vi "Verificacion_calibracion.vi"() -> ()   [LabVIEW 2015]
uses:
  <vilib>/LabVIEW Targets/FPGA/cRIO/shared/nicrio_ModuleControls/nicrio_cRIO-9234_DataRatesRing2.ctl
  <vilib>/userdefined/High Color/nirio_resource_hc.ctl
  <vilib>/Analysis/5stat.llb/RMS (DBL).vi
  <vilib>/Analysis/baseanly.llb/Mean (DBL).vi
  <vilib>/FPGAPlugInAG/cRIO-9031/niLvFpga_Open_cRIO-9031.vi
  <vilib>/FPGAPlugInAG/cRIO-9031/niLvFpga_Run_cRIO-9031.vi
  <vilib>/Utility/error.llb/Error Cluster From Error Code.vi
  <vilib>/rvi/errors/niLvFpgaAdjustHostInterfaceError.vi
  <vilib>/rvi/interface/common/niFpgaWaitOnOcc.vi
  <vilib>/FPGAPlugInAG/cRIO-9031/niLvFpga_Reset_cRIO-9031.vi
  <vilib>/measure/madcrms.llb/Basic Averaged DC-RMS for 1 Chan.vi
  <vilib>/measure/maspectr.llb/FFT Spectrum (Mag-Phase) for 1 Chan.vi
  <vilib>/FPGAPlugInAG/cRIO-9031/niLvFpga_Close_cRIO-9031.vi
  <vilib>/rvi/interface/nirviOpenFPGA/nirviOpenFPGA.xnode
  FPGA Bitfiles/WRDArabia_FPGATarget_FPGA8a2wsBIdirec_rZEOcJD8nrk.lvbitx
  <vilib>/rvi/interface/nirviMethod/nirviMethod.xnode
  <vilib>/rvi/interface/nirviReadWriteControl/nirviReadWriteControl.xnode
  <vilib>/rvi/interface/nirviCloseFPGA/nirviCloseFPGA.xnode
  <vilib>/measure/NI_MAPro.lvlib
  <vilib>/Analysis/NI_AALPro.lvlib
  <vilib>/Analysis/NI_AALBase.lvlib
  <vilib>/rvi/errors/niLvFpgaMergeErrorWithErrorCode.vi
  NiFpgaLv.dll
  <vilib>/FPGAPlugInAG/cRIO-9031/niLvFpga_ConfigureFifo_cRIO-9031.vi
  <vilib>/FPGAPlugInAG/cRIO-9031/niLvFpga_StartFifo_cRIO-9031.vi
  <vilib>/FPGAPlugInAG/cRIO-9031/niLvFpga_ReadFifo_cRIO-9031.vi
  <vilib>/FPGAPlugInAG/cRIO-9031/niLvFpga_StopFifo_cRIO-9031.vi
panel:
  out "size(s)":i32
  out "Numeric":i32
  in  "Pattern acceleration (g RMS)":dbl=1.0
  in  "Pattern frequency (Hz)":dbl=159.2
  out "RMS":dbl format="%0.2f"
  in  "Data Rate":T1=2 items=["51.200 kS/s (NI 9234)"=1, "25.600 kS/s (NI 9234)"=2, "17.067 kS/s (NI 9234)"=3, "12.800 kS/s (NI 9234)"=4, "10.240 kS/s (NI 9234)"=5, "8.533 kS/s (NI 9234)"=6, "7.314 kS/s (NI 9234)"=7, "6.400 kS/s (NI 9234)"=8, "5.689 kS/s (NI 9234)"=9, "5.120 kS/s (NI 9234)"=10, "4.654 kS/s (NI 9234)"=11, "4.267 kS/s (NI 9234)"=12, "3.938 kS/s (NI 9234)"=13, "3.657 kS/s (NI 9234)"=14, "3.413 kS/s (NI 9234)"=15, "3.200 kS/s (NI 9234)"=16, "3.012 kS/s (NI 9234)"=17, "2.845 kS/s (NI 9234)"=18, "2.695 kS/s (NI 9234)"=19, "2.560 kS/s (NI 9234)"=20, "2.438 kS/s (NI 9234)"=21, "2.328 kS/s (NI 9234)"=22, "2.226 kS/s (NI 9234)"=23, "2.133 kS/s (NI 9234)"=24, "2.048 kS/s (NI 9234)"=25, "1.969 kS/s (NI 9234)"=26, "1.896 kS/s (NI 9234)"=27, "1.829 kS/s (NI 9234)"=28, "1.765 kS/s (NI 9234)"=29, "1.707 kS/s (NI 9234)"=30, "1.652 kS/s (NI 9234)"=31]
  in  "Channel Nº":i32
  out "FREQUENCY SIGNAL":cluster{"f0":dbl, "df":dbl, "magnitude":dbl[]}(graph)
  out "error out":errorcluster
  out "Chassis \nTemperature":i16
  in  "Adquirir":bool
  out "Waveform Graph":waveform(dbl)[](graph)
  out "Frequency measured (Hz)":dbl
  in  "Sensivity Parameter\n           (mV/g)":sgl=10.0
  in  "Rate frequency (Hz)":dbl=25600.0
  in  "Calibration channels (4 o 8)":u32=8
  out "Nombre de archivo":path
  out "Tiempo de paso (s)":dbl
  in  "Acquisition time":dbl=1.0
  out "Buffer Overflow":bool
  out "Buffer Underflow":bool
  in  "stop":bool
  out "Inicio pasada":timestamp
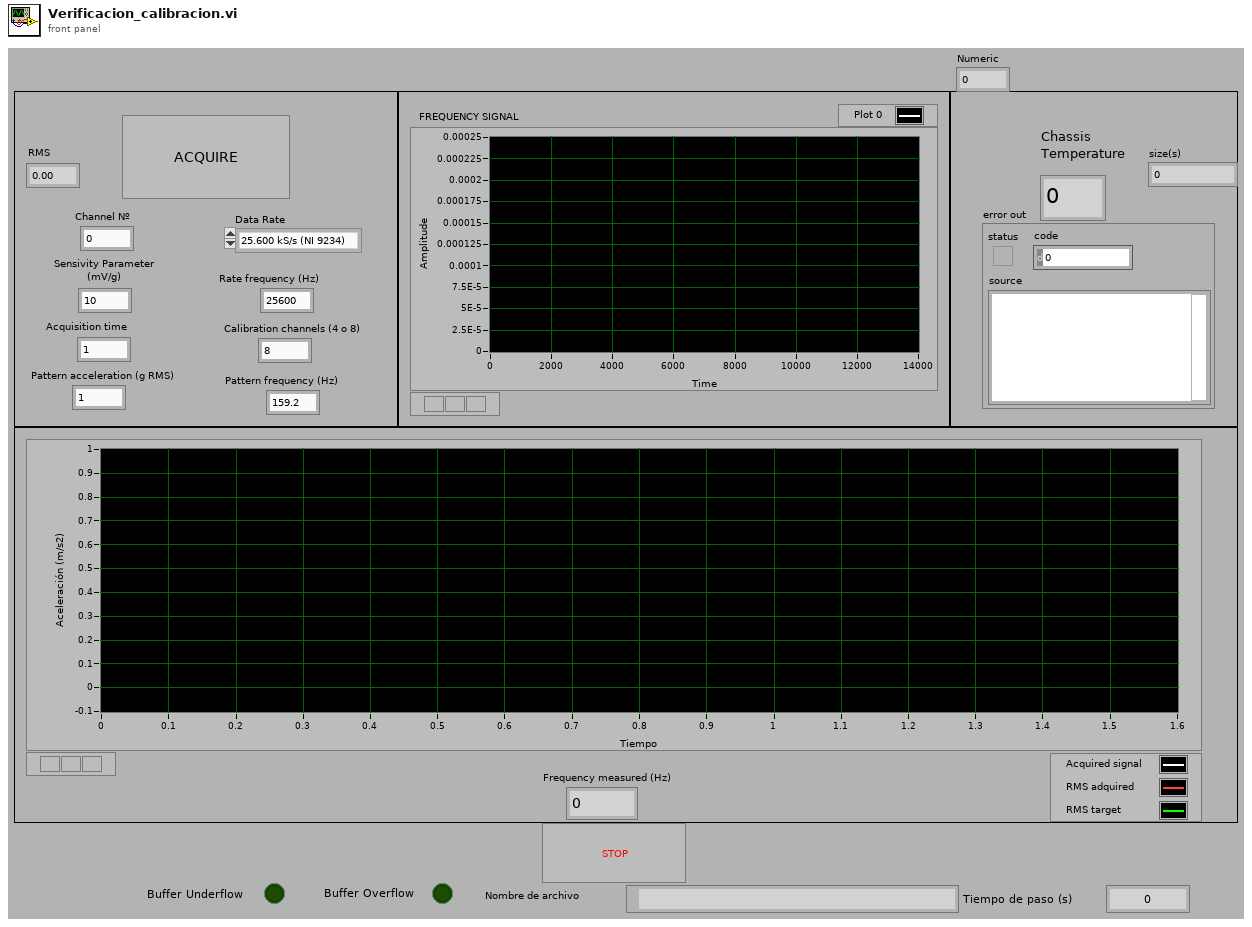
[diagram p1: front panel]
types:
  T1 = typedef "nicrio_cRIO-9234_DataRatesRing2.ctl" = u8
  T2 = typedef "nirio_resource_hc.ctl" = tag
  T3 = enum16{"open", "replace", "create", "open or create", "replace or create", "replace or create with confirmation"}
  T4 = enum16{"big-endian, network order", "native, host order", "little-endian"}
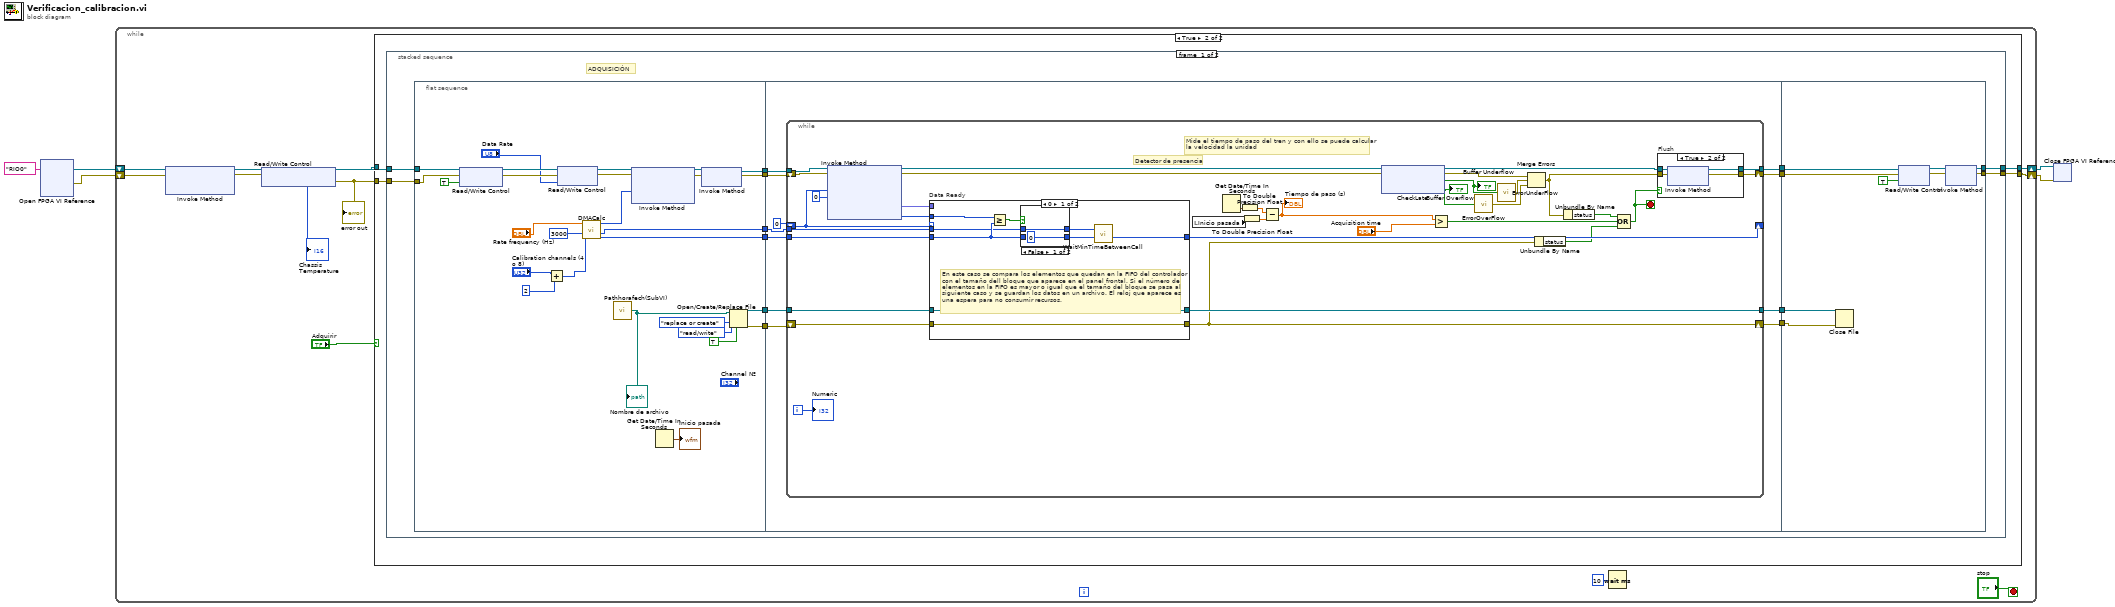
[diagram p0: block diagram]
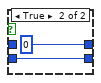
[diagram p3: hidden frame]
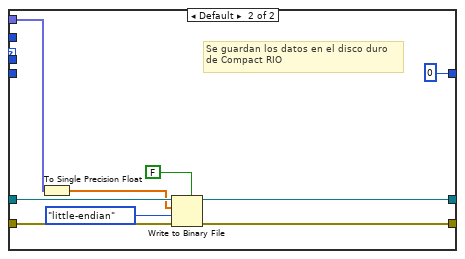
[diagram p4: hidden frame]
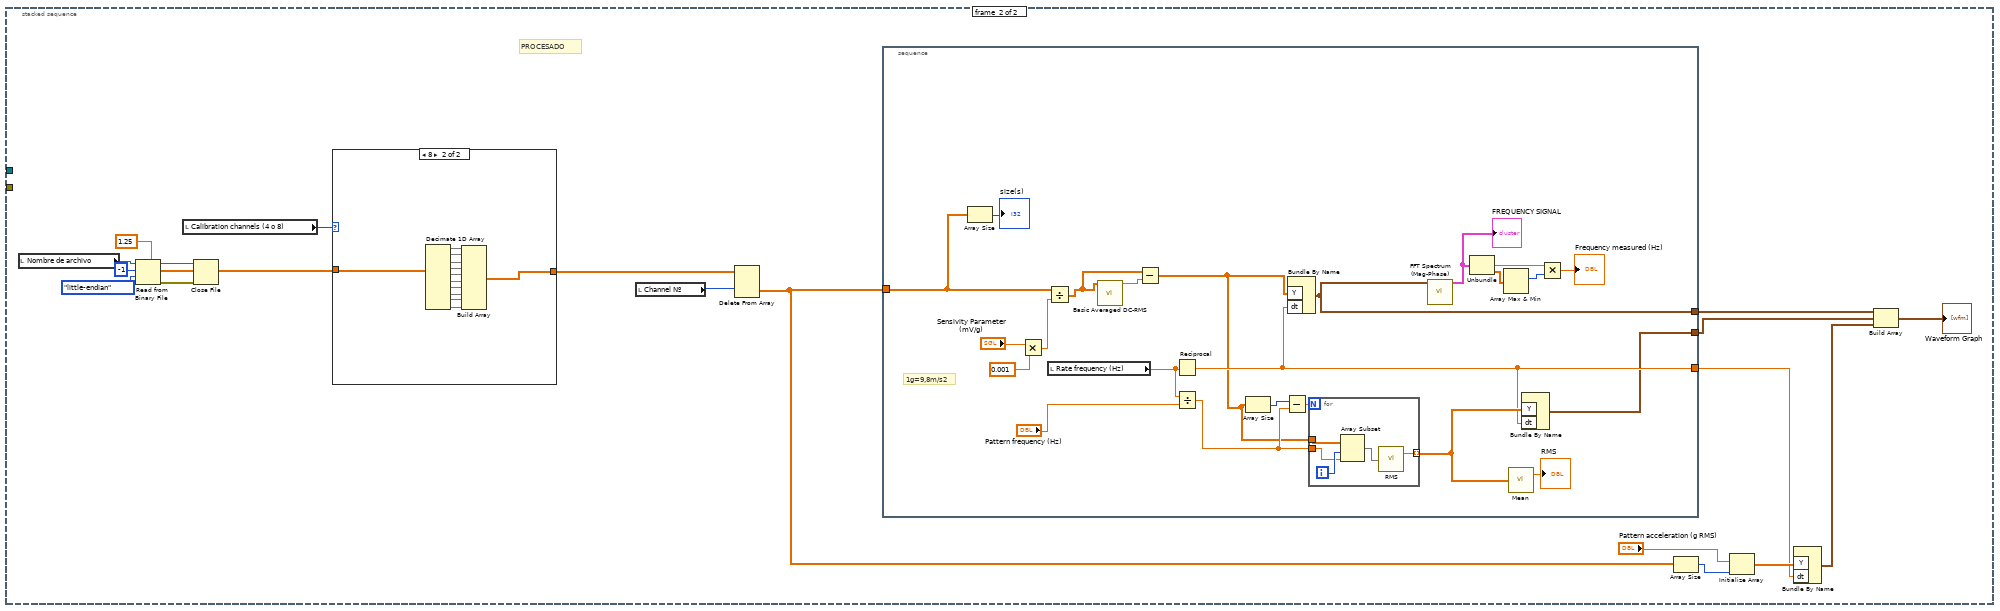
[diagram p6: hidden frame]
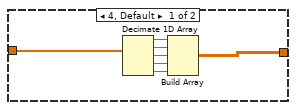
[diagram p7: hidden frame]
diagram:
  n1 = xnode "Open FPGA VI Reference"("resource name"=T2 "RIO0") -> ("FPGA VI Reference Out"=w5:refnum<k20>, "error out"=w2:errorcluster)  [unwired: 1 in]
  n2 = while {
    shift-right: [w10] -> w3
    shift-left: w5 -> [w8]
    shift-right: [w15] -> w4
    shift-left: w2 -> [w7]
    stop <- "stop" stop-if-true
    n3 = xnode "Invoke Method"("FPGA VI Reference In"=w8, "error in"=w7) -> ("FPGA VI Reference Out"=w9:refnum<k20>, "error out"=w6:errorcluster)  [unwired: 1 in]
    n4 = xnode "Read/Write Control"("FPGA VI Reference In"=w9, "error in"=w6) -> ("FPGA VI Reference Out"=w13:refnum<k20>, "error out"=w12:errorcluster, "Chassis Temperature"=→"Chassis \nTemperature":i16)
    "error out" <- w12
    n5 = case shown="True" "Adquirir" {
      tunnel: w13 -> [w19 w23]
      tunnel: w12 -> [w18 w22]
      tunnel: [w19 w21] -> w10
      tunnel: [w18 w20] -> w15
      frame False {
      }
      frame True {
        n6 = stacked-sequence {
          tunnel: w23 -> [w27 _]
          tunnel: w22 -> [w26 _]
          tunnel: [w25 _] -> w21
          tunnel: [w24 _] -> w20
          frame #0 {
            # "ADQUISICIÓN"
            n7 = flat-sequence {
              tunnel: w26 -> [w45]
              tunnel: w27 -> [w46]
              tunnel: [w57] -> w37
              tunnel: [w56] -> w36
              tunnel: [w55] -> w35
              tunnel: [w54] -> w34
              tunnel: [w53] -> w33
              tunnel: [w52] -> w32
              tunnel: [w74] -> w31
              tunnel: [w73] -> w30
              tunnel: [w72] -> w29
              tunnel: [w65] -> w28
              tunnel: w37 -> [w71]
              tunnel: w36 -> [w70]
              tunnel: w35 -> [w69]
              tunnel: w34 -> [w68]
              tunnel: w33 -> [w67]
              tunnel: w32 -> [w66]
              tunnel: w31 -> [w139]
              tunnel: w30 -> [w138]
              tunnel: w29 -> [w144]
              tunnel: w28 -> [w143]
              tunnel: [w145] -> w24
              tunnel: [w146] -> w25
              frame #0 {
                n8 = xnode "Read/Write Control"("FPGA VI Reference In"=w46, "error in"=w45, "Fotocélula"=TRUE ("Adquirir")) -> ("FPGA VI Reference Out"=w44:refnum<k20>, "error out"=w43:errorcluster)
                n9 = Add(x="Calibration channels (4 o 8)", y=u32 2) -> (x+y=w39:u32)
                n10 = xnode "Read/Write Control"("FPGA VI Reference In"=w44, "error in"=w43, "Data Rate"="Data Rate") -> ("FPGA VI Reference Out"=w50:refnum<k20>, "error out"=w49:errorcluster)
                n11 = call "DMACalc.vi"("Number of Channels"=w39, "Number of Samples"=u32 3000, "Rate (Hz)"="Rate frequency (Hz)") -> ("Block Size"=w54:u32, "Time to Acquire Block (ms)"=w55:i32, "Host Buffer Size"=w59:u32)  [unwired: 6 in]
                n12 = call "Pathhorafech(SubVI).vi"() -> ("path"=w58:path)
                "Nombre de archivo" <- w58
                n13 = xnode "Invoke Method"("FPGA VI Reference In"=w50, "error in"=w49, "Requested Depth"=w59) -> ("FPGA VI Reference Out"=w61:refnum<k20>, "error out"=w60:errorcluster)  [unwired: 1 out]
                n14 = Get Date/Time In Seconds() -> (seconds since 1Jan1904=→"Inicio pasada":timestamp)
                n15 = xnode "Invoke Method"("FPGA VI Reference In"=w61, "error in"=w60) -> ("FPGA VI Reference Out"=w57:refnum<k20>, "error out"=w56:errorcluster)
                n16 = Open/Create/Replace File(file path (use dialog)=w58, operation (0:open)=T3."replace or create", access (0:read/write)=enum16{"read/write", "read-only", "write-only"}."read/write", disable buffering (F)=TRUE) -> (refnum out=w53:refnum<file>, error out=w52:errorcluster)  [unwired: 1 in, 2 out]
              }
              frame #1 {
                n17 = while "Data Acquisition" {
                  tunnel: w71 -> [w101]
                  shift-right: [w108] -> _
                  shift-left: u32 0 ("t") -> [w104]
                  tunnel: w69 -> [w109]
                  tunnel: w68 -> [w107]
                  shift-right: [w110] -> w73
                  shift-left: w70 -> [w100]
                  tunnel: [w105] -> w74
                  tunnel: w67 -> [w88]
                  tunnel: [w89] -> w72
                  shift-right: [w87] -> w65
                  shift-left: w66 -> [w98]
                  i -> [w76]
                  stop <- w106 stop-if-true
                  # "Detector de presencia"
                  # "Mide el tiempo de paso del tren y con ello se puede calcular\nla velocidad la unidad"
                  n18 = xnode "Invoke Method"("FPGA VI Reference In"=w101, "error in"=w100, "Number of Elements"=w104, "Timeout (ms)"=0) -> ("FPGA VI Reference Out"=w86:refnum<k20>, "error out"=w85:errorcluster, "Data"=w99:fxp<+/-,24,4>[], "Elements Remaining"=w102:u32)
                  n19 = case "Data Ready" shown="0" w104 {
                    tunnel: w109 -> [w115 _]
                    tunnel: [w114 u32 0 ("t")] -> w108
                    tunnel: w107 -> [w116 _]
                    tunnel: w102 -> [w113 _]
                    tunnel: w99 -> [_ w126]
                    tunnel: w98 -> [w112 w128]
                    tunnel: [w112 w127] -> w87
                    tunnel: w88 -> [w111 w125]
                    tunnel: [w111 w124] -> w89
                    frame 0 {
                      # "En este caso se compara los elementos que quedan en la FIFO del controlador\ncon el tamaño dell bloque que aparece en el panel frontal. Si el número de\nelementos en la FIFO es mayor o igual que el tamaño del bloque se pasa al\nsiguiente caso y se guardan los datos en un archivo. El reloj que aparece es\nuna espera para no consumir recursos."
                      n20 = Greater Or Equal?(x=w113, y=w116) -> (x >= y?=w117:bool)
                      n21 = case shown="False" w117 {
                        tunnel: [u32 0 ("Block Size") w121] -> w114
                        tunnel: [w120 0 ("t")] -> w118
                        tunnel: w115 -> [w120 _]
                        tunnel: w116 -> [_ w121]
                        frame False {
                        }
                        frame True {
                        }
                      }
                      n22 = call "WaitMinTimeBetweenCall.vi"("Minimum ms between calls"=w118) -> ()  [unwired: 2 in]
                    }
                    frame Default {
                      # "Se guardan los datos en el disco duro\nde Compact RIO"
                      n23 = To Single Precision Float(number=w126) -> (single precision float=w123:sgl[])
                      n24 = Write to Binary File(file (use dialog)=w125, data=w123, error in=w128, 5:FALSE ("prepend array or string size? (T)"), 9:T4."little-endian" ("byte order (0:big-endian, network order)")) -> (refnum out=w124:refnum<file>, error out=w127:errorcluster)  [unwired: 2 out]
                    }
                  }
                  n25 = local read "Inicio pasada"() -> (w83:timestamp)
                  n26 = Get Date/Time In Seconds() -> (seconds since 1Jan1904=w82:timestamp)
                  n27 = To Double Precision Float(number=w82) -> (double precision float=w80:dbl)
                  n28 = To Double Precision Float(number=w83) -> (double precision float=w84:dbl)
                  n29 = Subtract(x=w80, y=w84) -> (x-y=w91:dbl)
                  "Tiempo de paso (s)" <- w91
                  n30 = xnode ("CheckLate")("FPGA VI Reference In"=w86, "error in"=w85) -> ("FPGA VI Reference Out"=w77:refnum<k20>, "error out"=w94:errorcluster, "Buffer Underflow"=w95:bool, "Buffer Overflow"=w96:bool)
                  "Buffer Underflow" <- w95
                  "Buffer Overflow" <- w96
                  n31 = Greater?(x=w91, y="Acquisition time") -> (0:w79:bool)
                  n32 = call "ErrorOverFlow.vi"("Buffer Overflow"=w96) -> ("error out"=w92:errorcluster)
                  n33 = call "ErrorUnderFlow.vi"("Buffer Overflow"=w95) -> ("error out"=w93:errorcluster)
                  n34 = Merge Errors(w94, w93, w92) -> (w78:errorcluster)
                  n35 = Unbundle By Name(w87) -> ("status"=w90:bool)
                  n36 = Unbundle By Name(w78) -> ("status"=w97:bool)
                  n37 = Compound Arithmetic op=OR(w97, w79, w90) -> (w106:bool)
                  n38 = case "Flush" shown="True" w106 {
                    tunnel: w77 -> [w132 w137]
                    tunnel: w78 -> [w133 w136]
                    tunnel: [w133 w135] -> w110
                    tunnel: [w132 w134] -> w105
                    frame False {
                    }
                    frame True {
                      n39 = xnode "Invoke Method"("FPGA VI Reference In"=w137, "error in"=w136) -> ("FPGA VI Reference Out"=w134:refnum<k20>, "error out"=w135:errorcluster)
                    }
                  }
                  "Numeric" <- w76
                }
              }
              frame #2 {
                n40 = Close File(refnum=w144, error in=w143) -> ()  [unwired: 2 out]
                n41 = xnode "Read/Write Control"("FPGA VI Reference In"=w139, "error in"=w138, "Stop"=TRUE ("stop")) -> ("FPGA VI Reference Out"=w142:refnum<k20>, "error out"=w141:errorcluster)
                n42 = xnode "Invoke Method"("FPGA VI Reference In"=w142, "error in"=w141) -> ("FPGA VI Reference Out"=w146:refnum<k20>, "error out"=w145:errorcluster)
              }
            }
          }
          frame #1 {
            # "PROCESADO"
            n43 = local read "Nombre de archivo"() -> (w162:path)
            n44 = Read from Binary File(5:sgl 1.25, 9:T4."little-endian" ("byte order (0:big-endian, network order)"), 10:-1 ("count (1)"), 11:w162) -> (0:w165:errorcluster, 2:w158:sgl[], 3:w161:refnum<file>)  [unwired: 1 in, 2 out]
            n45 = local read "Calibration channels (4 o 8)"() -> (w159:u32)
            n46 = Close File(refnum=w161, error in=w165) -> ()  [unwired: 2 out]
            n47 = case shown="8" w159 {
              tunnel: w158 -> [w197 w209]
              tunnel: [w196 w208] -> w157
              frame 4, Default {
                n48 = Decimate 1D Array(w197) -> (w199:sgl[], w200:sgl[], w198:sgl[], w195:sgl[], w194:sgl[])
                n49 = Build Array(w199, w200, w198, w195, w194) -> (w196:sgl[][])
              }
              frame 8 {
                n50 = Decimate 1D Array(w209) -> (w211:sgl[], w212:sgl[], w210:sgl[], w204:sgl[], w203:sgl[], w205:sgl[], w206:sgl[], w207:sgl[], w202:sgl[], w201:sgl[])
                n51 = Build Array(w211, w212, w210, w204, w203, w205, w206, w207, w202, w201) -> (w208:sgl[][])
              }
            }
            n52 = local read "Channel Nº"() -> (w156:i32)
            n53 = Delete From Array(array=w157, index (row)=w156) -> (deleted portion=w150:sgl[])  [unwired: 2 in, 1 out]
            n54 = stacked-sequence {
              tunnel: [w181] -> w155
              tunnel: [w170] -> w152
              tunnel: w150 -> [w167]
              tunnel: [w168] -> w147
              frame #0 {
                # "1g=9,8m/s2"
                n55 = Array Size(array=w167) -> (size(s)=→"size(s)":i32)
                n56 = Multiply(x="Sensivity Parameter\n           (mV/g)", y=0.001) -> (x*y=w183:dbl)
                n57 = Divide(x=w167, y=w183) -> (x/y=w178:dbl[])
                n58 = local read "Rate frequency (Hz)"() -> (w172:dbl)
                n59 = call-poly <vilib>:"Basic Averaged DC-RMS.vi"("signal in"=w178) -> ("DC value"=w180:dbl)  [unwired: 7 in, 3 out]
                n60 = Subtract(x=w178, y=w180) -> (x-y=w169:dbl[])
                n61 = Reciprocal(x=w172) -> (1/x=w170:dbl)
                n62 = Divide(x=w172, y="Pattern frequency (Hz)") -> (x/y=w175:dbl)
                n63 = Array Size(array=w169) -> (size(s)=w176:i32)
                n64 = Subtract(x=w176, y=w175) -> (x-y=w177:dbl)
                n65 = Bundle By Name("Y"=w169, "dt"=w170) -> (w181:waveform(dbl))  [unwired: 1 in]
                n66 = for {
                  N: w177 -> [_]
                  tunnel: w175 -> [w190]
                  tunnel: [w193] -> w174 mode=indexing
                  tunnel: w169 -> [w192]
                  i -> [w191]
                  n67 = Array Subset(array=w192, index=w191, length=w190) -> (w189:dbl[])
                  n68 = call-poly <vilib>:"RMS.vi"("X"=w189) -> ("rms value"=w193:dbl)  [unwired: 1 out]
                }
                n69 = call-poly <vilib>:"FFT Spectrum (Mag-Phase).vi"("time signal"=w181) -> ("magnitude"=w184:cluster{"f0":dbl, "df":dbl, "magnitude":dbl[]})  [unwired: 6 in, 4 out]
                "FREQUENCY SIGNAL" <- w184
                n70 = Unbundle(w184) -> ("df"=w186:dbl, "magnitude"=w187:dbl[])  [unwired: 1 out]
                n71 = Array Max & Min(array=w187) -> (max index (indices)=w188:i32)  [unwired: 3 out]
                n72 = call-poly <vilib>:"Mean.vi"("X"=w174) -> ("mean"=→"RMS":dbl)  [unwired: 1 out]
                n73 = Bundle By Name("Y"=w174, "dt"=w170) -> (w168:waveform(dbl))  [unwired: 1 in]
                n74 = Multiply(x=w186, y=w188) -> (x*y=→"Frequency measured (Hz)":dbl)
              }
            }
            n75 = Array Size(array=w150) -> (size(s)=w154:i32)
            n76 = Initialize Array("Pattern acceleration (g RMS)", w154) -> (w153:dbl[])
            n77 = Bundle By Name("Y"=w153, "dt"=w152) -> (w149:waveform(dbl))  [unwired: 1 in]
            n78 = Build Array(w155, w147, w149) -> (→"Waveform Graph":waveform(dbl)[])
          }
        }
      }
    }
    n79 = Wait (ms)(milliseconds to wait=u32 10) -> ()  [unwired: 1 out]
  }
  n80 = xnode "Close FPGA VI Reference"("FPGA VI Reference In"=w3, "error in"=w4) -> ()  [unwired: 1 out]
